vi "Compressor.vi"   [LabVIEW 2014]
uses:
  <vilib>/Rock Robotics/WPI/DriverStation/WPI_DriverStationRobotMode2.ctl
  Begin/Global Variables.vi
  Begin/Global RefNums.vi
  <vilib>/Rock Robotics/WPI/Compressor/WPI_CompressorGetSetRefNum.vi
types:
  T1 = typedef "WPI_DriverStationRobotMode2.ctl" = enum16{"Autonomous Disabled", "Autonomous Enabled", "Teleop Disabled", "Teleop Enabled", "Disconnected", "Finish", "Test Disabled", "Test Enabled", "Emergency Stopped"}
  T2 = typedef "WPI_CompressorDevRef.ctl" = cluster{"DevStatus":errorcluster, "Pneumatics Control Module":u8}
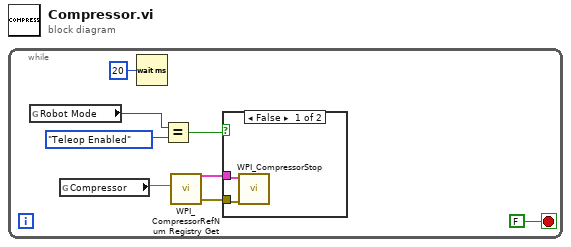
[diagram p0: block diagram]
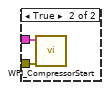
[diagram p2: hidden frame]
diagram:
  n1 = while {
    stop <- FALSE stop-if-true
    n2 = global read "Global Variables.vi" "Robot Mode"() -> (w8:T1)
    n3 = global read "Global RefNums.vi" "Compressor"() -> (w3:string)
    n4 = Wait (ms)(milliseconds to wait=u32 20) -> ()  [unwired: 1 out]
    n5 = Equal?(x=w8, y=WPI_DriverStationRobotMode2."Teleop Enabled") -> (x = y?=w6:bool)
    n6 = call <vilib>:"WPI_CompressorRefNum Registry Get.vi"("refnum name"=w3) -> ("error out"=w1:errorcluster, "CompressorDevRef"=w2:T2)  [unwired: 9 in]
    n7 = case shown="False" w6 {
      tunnel: w2 -> [w10 w12]
      tunnel: w1 -> [w9 w11]
      frame False {
        n8 = call <vilib>:"WPI_CompressorStop.vi"("error in (no error)"=w9, "CompressorDevRef"=w10) -> ()  [unwired: 8 in, 2 out]
      }
      frame True {
        n9 = call <vilib>:"WPI_CompressorStart.vi"("error in (no error)"=w11, "CompressorDevRef"=w12) -> ()  [unwired: 8 in, 2 out]
      }
    }
  }
